vi "텍스트링.vi"() -> ()   [LabVIEW 2019]
panel:
  in  "Ring":u16(ring) items=["일"=65535, "시간"=3600, "분"=60, "초"=1, ""=0]
  out "초단위":dbl
  in  "시간입력":dbl
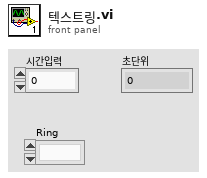
[diagram p1: front panel]
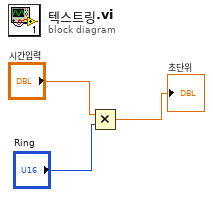
[diagram p0: block diagram]
diagram:
  n1 = Multiply(x="시간입력", y="Ring") -> (x*y=→"초단위":dbl)
